vi "PathChecker.vi"() -> ()   [LabVIEW 2025]
panel:
  out "Table Control":string[][](table)
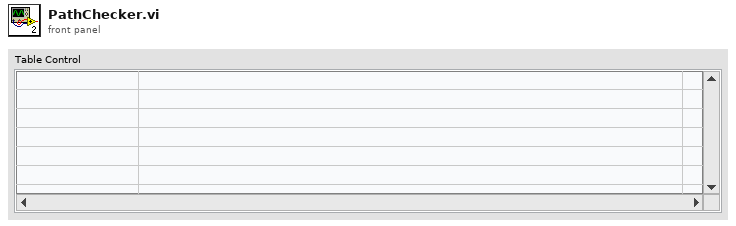
[diagram p1: front panel]
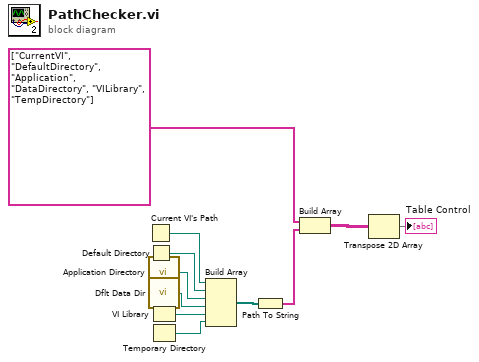
[diagram p0: block diagram]
diagram:
  n1 = Current VI's Path() -> (path=w11:path)
  n2 = Default Directory() -> (w10:path)
  n3 = call <vilib>:"Application Directory.vi"() -> ("Application Directory"=w9:path)
  n4 = call <vilib>:"Dflt Data Dir.vi"() -> ("App:Default Data Directory"=w8:path)
  n5 = VI Library() -> (path=w7:path)
  n6 = Temporary Directory() -> (w6:path)
  n7 = Build Array(w11, w10, w9, w8, w7, w6) -> (w5:path[])
  n8 = Path To String(path=w5) -> (string=w4:string[])
  n9 = Build Array(string[] ["CurrentVI", "DefaultDirectory", "Application", "DataDirectory", "VILibrary", "TempDirectory"], w4) -> (w2:string[][])
  n10 = Transpose 2D Array(2D array=w2) -> (transposed array=→"Table Control":string[][])
